vi "OPC.vi"() -> ()   [LabVIEW 2015]
uses:
  <vilib>/Platform/TimedLoop/XDataNode/timing_clust.ctl
  <vilib>/Platform/TimedLoop/XDataNode/nitl_modes.ctl
  <vilib>/Platform/TimedLoop/XDataNode/wakeup.ctl
  Global control/global-opc.vi
  <vilib>/Platform/TimedLoop/XDataNode/XDataNode.xnode
  <vilib>/Platform/TimedLoop/XDataNode/XDNodeRunTimeDep.lvlib
panel:
  out "IP40":T1={"toHMI正常运行"=TRUE, "toHMI设备准备好"=TRUE, "toHMI设备异常"=TRUE, "toHMI刀开关分—状态"=TRUE, "toHMI刀开关合—状态"=TRUE, "toHMI框架电流故障"=TRUE, "toHMI框架电压故障"=TRUE, "toHMII段电压故障"=TRUE, "toHMIII段电压故障"=TRUE, "toHMI装置故障"=TRUE, "toHMIMCB故障"=TRUE, "toHMI刀开关合—完成"=TRUE, "toHMI复位按钮"=TRUE, "toHMI远程"=TRUE, "toHMI本地"=TRUE, "模拟电流框架故障控制"=TRUE, "模拟电压框架故障控制"=TRUE, "模拟I段电压故障控制"=TRUE, "模拟II段电压故障控制"=TRUE, "故障复位控制"=TRUE}
  out "IP30":T2={"toHMI正常运行"=FALSE, "toHMI设备准备好"=FALSE, "toHMI设备异常"=FALSE, "toHMI高断分—状态"=FALSE, "toHMI高断合—状态"=FALSE, "toHMI继保故障信号"=FALSE, "toHMI远方"=FALSE, "toHMI本地"=FALSE, "toHMI旁路合闸—按钮"=FALSE, "toHMI旁路分闸—按钮"=FALSE, "toHMI允许高断合闸—状态"=FALSE, "toHMI旁路合分闸—状态"=FALSE, "1500V电压输出"=0, "高断储能控制"=TRUE, "旁路合闸控制"=TRUE, "旁路分闸控制"=TRUE}
  out "IP20":T3={"toHMI正常运行"=TRUE, "toHMI设备准备好"=TRUE, "toHMI设备异常"=TRUE, "toHMI刀开关合—状态"=TRUE, "toHMI刀开关分—状态"=TRUE, "toHMI刀开关合按钮"=TRUE, "toHMI刀开关分按钮"=TRUE, "toHMI复位按钮"=TRUE, "toHMI远程"=TRUE, "toHMI本地"=TRUE, "toHMI刀闸合—动作"=TRUE, "toHMI刀闸分—动作"=TRUE, "刀开关合闸控制"=TRUE, "刀开关分闸控制"=TRUE, "故障复位控制"=TRUE}
  out "IP10":T4
  out "IP50":T5={"toHMI刀开关合—状态"=TRUE, "toHMI刀开关分—状态"=TRUE, "toHMI刀开关合按钮"=TRUE, "toHMI刀开关分按钮"=TRUE, "toHMI远程"=TRUE, "toHMI本地"=TRUE, "toHMI正常运行"=TRUE, "toHMI设备准备好"=TRUE, "toHMI设备异常"=TRUE, "toHMI刀闸合—动作"=TRUE, "toHMI刀闸分—动作"=TRUE, "toHMI接触轨有压"=TRUE, "刀开关合闸控制"=TRUE, "刀开关分闸控制"=TRUE}
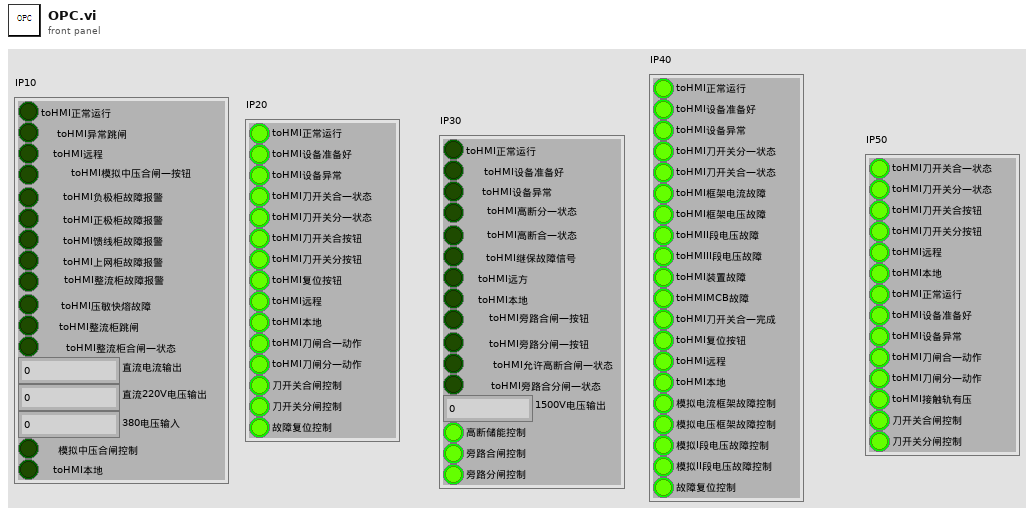
[diagram p1: front panel]
types:
  T1 = cluster{"toHMI正常运行":bool, "toHMI设备准备好":bool, "toHMI设备异常":bool, "toHMI刀开关分—状态":bool, "toHMI刀开关合—状态":bool, "toHMI框架电流故障":bool, "toHMI框架电压故障":bool, "toHMII段电压故障":bool, "toHMIII段电压故障":bool, "toHMI装置故障":bool, "toHMIMCB故障":bool, "toHMI刀开关合—完成":bool, "toHMI复位按钮":bool, "toHMI远程":bool, "toHMI本地":bool, "模拟电流框架故障控制":bool, "模拟电压框架故障控制":bool, "模拟I段电压故障控制":bool, "模拟II段电压故障控制":bool, "故障复位控制":bool}
  T2 = cluster{"toHMI正常运行":bool, "toHMI设备准备好":bool, "toHMI设备异常":bool, "toHMI高断分—状态":bool, "toHMI高断合—状态":bool, "toHMI继保故障信号":bool, "toHMI远方":bool, "toHMI本地":bool, "toHMI旁路合闸—按钮":bool, "toHMI旁路分闸—按钮":bool, "toHMI允许高断合闸—状态":bool, "toHMI旁路合分闸—状态":bool, "1500V电压输出":u32, "高断储能控制":bool, "旁路合闸控制":bool, "旁路分闸控制":bool}
  T3 = cluster{"toHMI正常运行":bool, "toHMI设备准备好":bool, "toHMI设备异常":bool, "toHMI刀开关合—状态":bool, "toHMI刀开关分—状态":bool, "toHMI刀开关合按钮":bool, "toHMI刀开关分按钮":bool, "toHMI复位按钮":bool, "toHMI远程":bool, "toHMI本地":bool, "toHMI刀闸合—动作":bool, "toHMI刀闸分—动作":bool, "刀开关合闸控制":bool, "刀开关分闸控制":bool, "故障复位控制":bool}
  T4 = cluster{"toHMI正常运行":bool, "toHMI异常跳闸":bool, "toHMI远程":bool, "toHMI模拟中压合闸—按钮":bool, "toHMI负极柜故障报警":bool, "toHMI正极柜故障报警":bool, "toHMI馈线柜故障报警":bool, "toHMI上网柜故障报警":bool, "toHMI整流柜故障报警":bool, "toHMI压敏快熔故障":bool, "toHMI整流柜跳闸":bool, "toHMI整流柜合闸—状态":bool, "直流电流输出":u32, "直流220V电压输出":u32, "380电压输入":u32, "模拟中压合闸控制":bool, "toHMI本地":bool}
  T5 = cluster{"toHMI刀开关合—状态":bool, "toHMI刀开关分—状态":bool, "toHMI刀开关合按钮":bool, "toHMI刀开关分按钮":bool, "toHMI远程":bool, "toHMI本地":bool, "toHMI正常运行":bool, "toHMI设备准备好":bool, "toHMI设备异常":bool, "toHMI刀闸合—动作":bool, "toHMI刀闸分—动作":bool, "toHMI接触轨有压":bool, "刀开关合闸控制":bool, "刀开关分闸控制":bool}
  T6 = typedef "XDNodeRunTimeDep.lvlib/timing_clust.ctl" = cluster{"Expected End [f-1]":u64, "Actual End [f-1]":u64, "Finished Late? [f-1]":bool, "Expected End [i-1]":u64, "Actual End [i-1]":u64, "Finished Late? [i-1]":bool, "Expected Start [i]":u64, "Actual Start [i]":u64, "Expected Start [f]":u64, "Actual Start [f]":u64, "Source Name":string, "Structure Name":string, "Period":i64, "Deadline":i64, "Offset":i64, "Start":i64, "Priority":i32, "Timeout":i32, "Mode":T7, "Wakeup Reason":T8, "Error":errorcluster, "Source Type":string, "Secondary Source Type":string, "Global End Time":u64, "Global Start Time":u64, "Frame Duration":u64, "Iteration Duration":u64, "Assigned CPU":i32, "I/O Scan Engine Mode":u32}
  T7 = typedef "XDNodeRunTimeDep.lvlib/nitl_modes.ctl" = enum32{"No Change", "Process missed periods, maintain original phase", "Discard missed periods, maintain original phase", "Process missed periods, ignore original phase", "Discard missed periods, ignore original phase"}
  T8 = typedef "XDNodeRunTimeDep.lvlib/wakeup.ctl" = enum32{"Normal", "Aborted", "Asynchronous wakeup", "Timing source error", "Timed loop error", "Timeout"}
  T9 = cluster{bool, bool, bool, bool, bool, bool, bool, bool, bool, bool, bool, bool, bool, bool, bool}
  T10 = cluster{bool, bool, bool, bool, bool, bool, bool, bool, bool, bool, bool, bool, u32, bool, bool, bool}
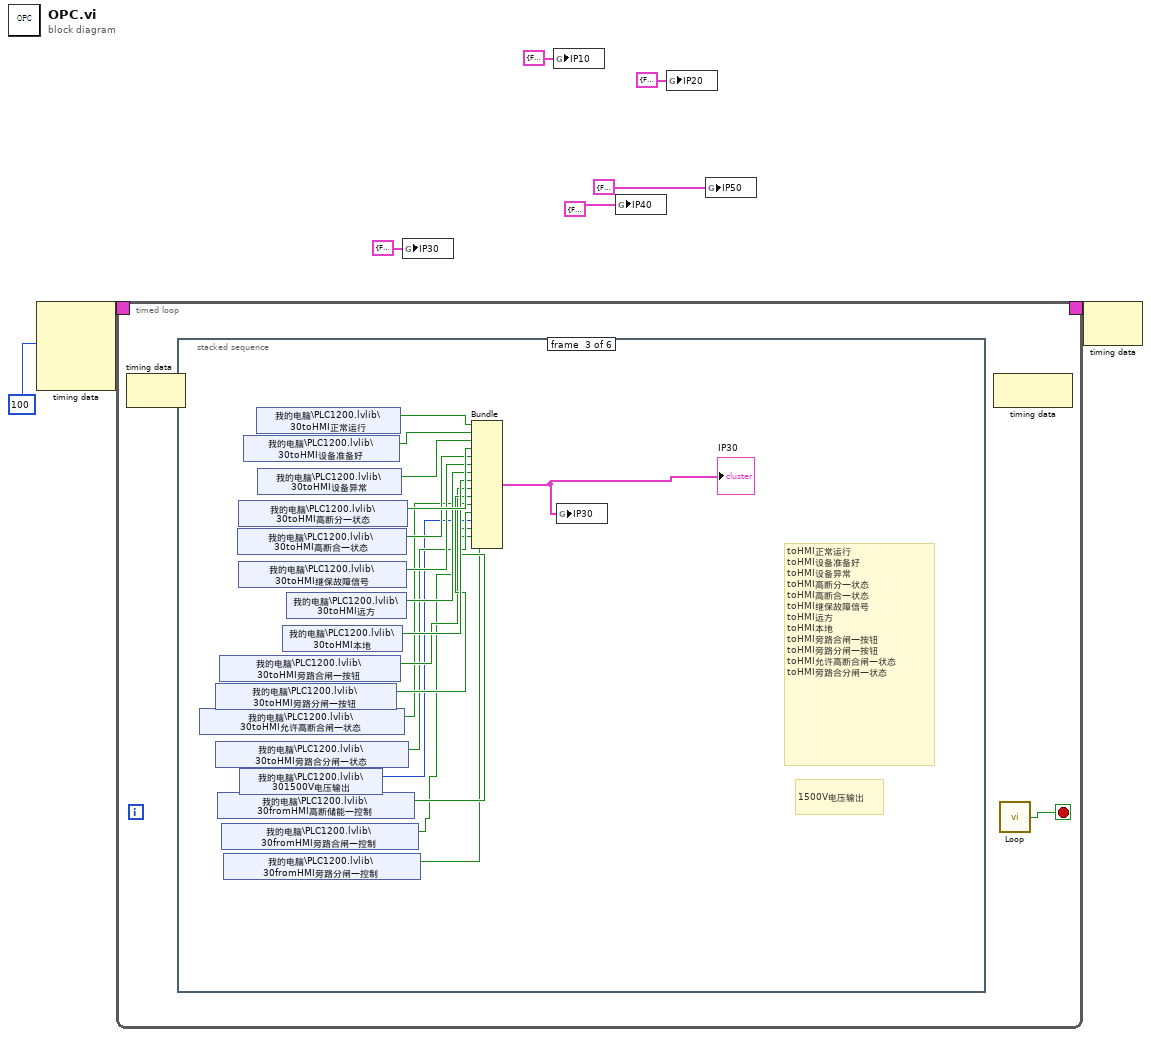
[diagram p0: block diagram]
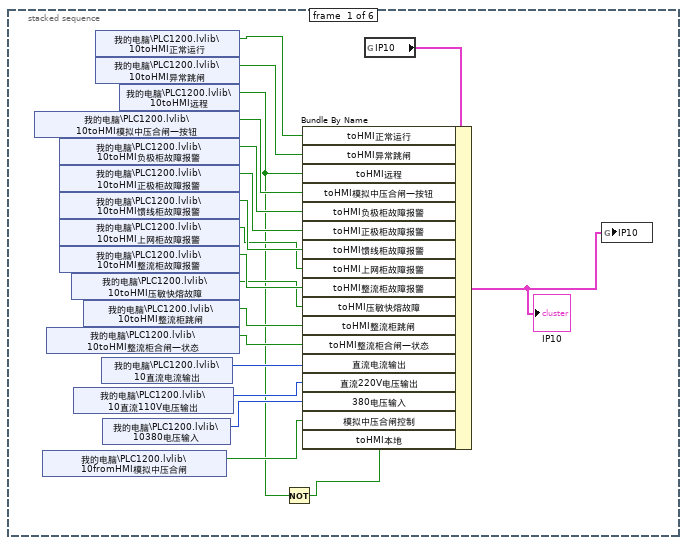
[diagram p2: hidden frame]
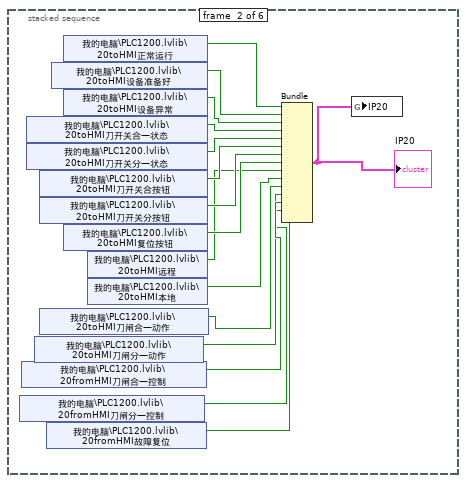
[diagram p3: hidden frame]
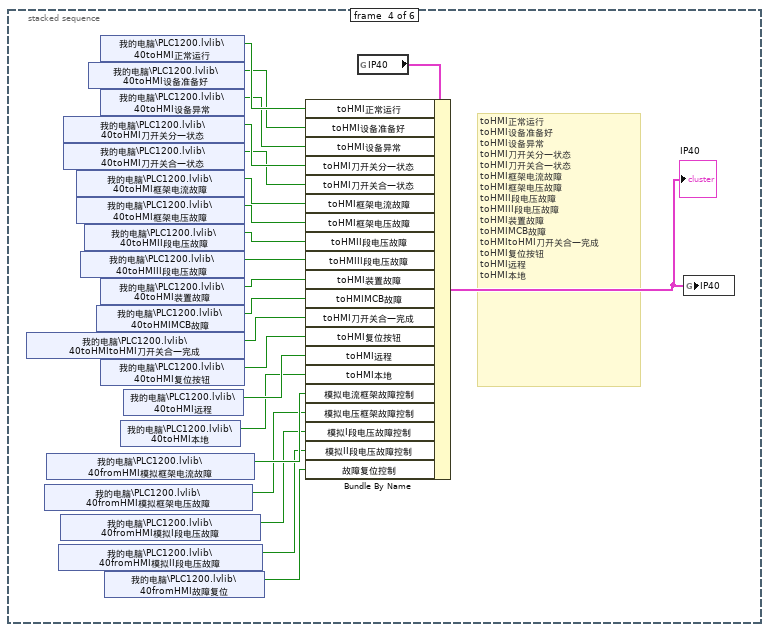
[diagram p4: hidden frame]
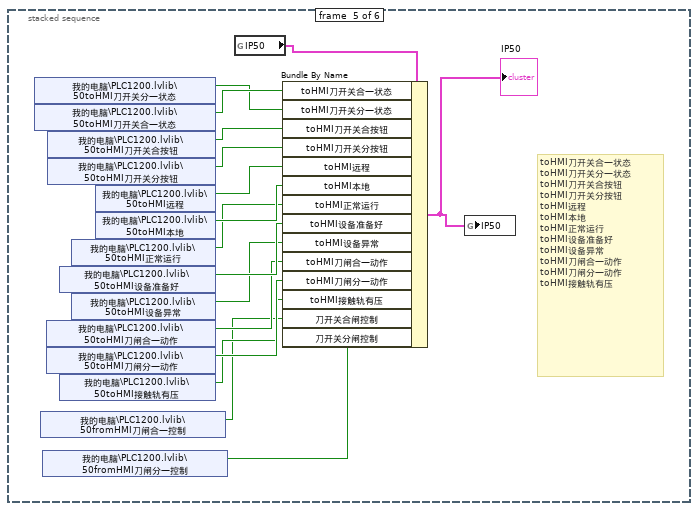
[diagram p5: hidden frame]
diagram:
  n1 = node-c288(i64 100 ("周期")) -> (w8:T6)  [unwired: 3 in]
  n2 = timed-loop {
    timing: w8 -> [_]
    timing-out: [_] -> w7
    stop <- w9 stop-if-true
    # "IP192.168.0.10"
    n3 = node-c288() -> ()  [unwired: 1 in, 1 out]
    n4 = stacked-sequence {
      frame #0 {
        n5 = shared-variable "我的电脑\\PLC1200.lvlib\\10toHMI模拟中压合闸—按钮"() -> (w25:bool)  [unwired: 1 in, 1 out]
        n6 = shared-variable "我的电脑\\PLC1200.lvlib\\10fromHMI模拟中压合闸"() -> (w13:bool)  [unwired: 1 in, 1 out]
        n7 = shared-variable "我的电脑\\PLC1200.lvlib\\10toHMI整流柜合闸—状态"() -> (w17:bool)  [unwired: 1 in, 1 out]
        n8 = shared-variable "我的电脑\\PLC1200.lvlib\\10toHMI负极柜故障报警"() -> (w24:bool)  [unwired: 1 in, 1 out]
        n9 = shared-variable "我的电脑\\PLC1200.lvlib\\10toHMI正极柜故障报警"() -> (w23:bool)  [unwired: 1 in, 1 out]
        n10 = shared-variable "我的电脑\\PLC1200.lvlib\\10toHMI馈线柜故障报警"() -> (w22:bool)  [unwired: 1 in, 1 out]
        n11 = shared-variable "我的电脑\\PLC1200.lvlib\\10toHMI上网柜故障报警"() -> (w21:bool)  [unwired: 1 in, 1 out]
        n12 = shared-variable "我的电脑\\PLC1200.lvlib\\10toHMI整流柜故障报警"() -> (w20:bool)  [unwired: 1 in, 1 out]
        n13 = shared-variable "我的电脑\\PLC1200.lvlib\\10toHMI压敏快熔故障"() -> (w19:bool)  [unwired: 1 in, 1 out]
        n14 = shared-variable "我的电脑\\PLC1200.lvlib\\10直流110V电压输出"() -> (w15:u32)  [unwired: 1 in, 1 out]
        n15 = shared-variable "我的电脑\\PLC1200.lvlib\\10toHMI整流柜跳闸"() -> (w18:bool)  [unwired: 1 in, 1 out]
        n16 = shared-variable "我的电脑\\PLC1200.lvlib\\10toHMI正常运行"() -> (w27:bool)  [unwired: 1 in, 1 out]
        n17 = shared-variable "我的电脑\\PLC1200.lvlib\\10toHMI异常跳闸"() -> (w26:bool)  [unwired: 1 in, 1 out]
        n18 = shared-variable "我的电脑\\PLC1200.lvlib\\10直流电流输出"() -> (w16:u32)  [unwired: 1 in, 1 out]
        n19 = shared-variable "我的电脑\\PLC1200.lvlib\\10380电压输入"() -> (w14:u32)  [unwired: 1 in, 1 out]
        n20 = shared-variable "我的电脑\\PLC1200.lvlib\\10toHMI远程"() -> (w11:bool)  [unwired: 1 in, 1 out]
        n21 = Not(x=w11) -> (.not. x?=w10:bool)
        n22 = global read "global-opc.vi" "IP10"() -> (w28:T4)
        n23 = Bundle By Name(cluster=w28, "toHMI正常运行"=w27, "toHMI异常跳闸"=w26, "toHMI远程"=w11, "toHMI模拟中压合闸—按钮"=w25, "toHMI负极柜故障报警"=w24, "toHMI正极柜故障报警"=w23, "toHMI馈线柜故障报警"=w22, "toHMI上网柜故障报警"=w21, "toHMI整流柜故障报警"=w20, "toHMI压敏快熔故障"=w19, "toHMI整流柜跳闸"=w18, "toHMI整流柜合闸—状态"=w17, "直流电流输出"=w16, "直流220V电压输出"=w15, "380电压输入"=w14, "模拟中压合闸控制"=w13, "toHMI本地"=w10) -> (w12:T4)
        "IP10" <- w12
        n24 = global write "global-opc.vi" "IP10"(w12) -> ()
      }
      frame #1 {
        n25 = shared-variable "我的电脑\\PLC1200.lvlib\\20fromHMI刀闸分—控制"() -> (w32:bool)  [unwired: 1 in, 1 out]
        n26 = shared-variable "我的电脑\\PLC1200.lvlib\\20fromHMI刀闸合—控制"() -> (w33:bool)  [unwired: 1 in, 1 out]
        n27 = shared-variable "我的电脑\\PLC1200.lvlib\\20toHMI刀开关合—状态"() -> (w44:bool)  [unwired: 1 in, 1 out]
        n28 = shared-variable "我的电脑\\PLC1200.lvlib\\20toHMI刀开关分—状态"() -> (w43:bool)  [unwired: 1 in, 1 out]
        n29 = shared-variable "我的电脑\\PLC1200.lvlib\\20toHMI刀闸分—动作"() -> (w30:bool)  [unwired: 1 in, 1 out]
        n30 = shared-variable "我的电脑\\PLC1200.lvlib\\20toHMI刀开关合按钮"() -> (w42:bool)  [unwired: 1 in, 1 out]
        n31 = shared-variable "我的电脑\\PLC1200.lvlib\\20toHMI刀开关分按钮"() -> (w41:bool)  [unwired: 1 in, 1 out]
        n32 = shared-variable "我的电脑\\PLC1200.lvlib\\20toHMI刀闸合—动作"() -> (w29:bool)  [unwired: 1 in, 1 out]
        n33 = shared-variable "我的电脑\\PLC1200.lvlib\\20fromHMI故障复位"() -> (w31:bool)  [unwired: 1 in, 1 out]
        n34 = shared-variable "我的电脑\\PLC1200.lvlib\\20toHMI设备准备好"() -> (w36:bool)  [unwired: 1 in, 1 out]
        n35 = shared-variable "我的电脑\\PLC1200.lvlib\\20toHMI正常运行"() -> (w37:bool)  [unwired: 1 in, 1 out]
        n36 = shared-variable "我的电脑\\PLC1200.lvlib\\20toHMI设备异常"() -> (w35:bool)  [unwired: 1 in, 1 out]
        n37 = shared-variable "我的电脑\\PLC1200.lvlib\\20toHMI复位按钮"() -> (w40:bool)  [unwired: 1 in, 1 out]
        n38 = shared-variable "我的电脑\\PLC1200.lvlib\\20toHMI远程"() -> (w39:bool)  [unwired: 1 in, 1 out]
        n39 = shared-variable "我的电脑\\PLC1200.lvlib\\20toHMI本地"() -> (w38:bool)  [unwired: 1 in, 1 out]
        n40 = Bundle(w37, w36, w35, w44, w43, w42, w41, w40, w39, w38, w29, w30, w33, w32, w31) -> (w34:T9)  [unwired: 1 in]
        "IP20" <- w34
        n41 = global write "global-opc.vi" "IP20"(w34) -> ()
      }
      frame #2 {
        # "1500V电压输出"
        # "toHMI正常运行\ntoHMI设备准备好\ntoHMI设备异常\ntoHMI高断分—状态\ntoHMI高断合—状态\ntoHMI继保故障信号\ntoHMI远方\ntoHMI本地\ntoHMI旁路合闸—按钮\ntoHMI旁路分闸—按钮\ntoHMI允许高断合闸—状态\ntoHMI旁路合分闸—状态"
        n42 = shared-variable "我的电脑\\PLC1200.lvlib\\30toHMI允许高断合闸—状态"() -> (w51:bool)  [unwired: 1 in, 1 out]
        n43 = shared-variable "我的电脑\\PLC1200.lvlib\\30toHMI旁路分闸—按钮"() -> (w53:bool)  [unwired: 1 in, 1 out]
        n44 = shared-variable "我的电脑\\PLC1200.lvlib\\30toHMI旁路合分闸—状态"() -> (w50:bool)  [unwired: 1 in, 1 out]
        n45 = shared-variable "我的电脑\\PLC1200.lvlib\\30fromHMI高断储能—控制"() -> (w47:bool)  [unwired: 1 in, 1 out]
        n46 = shared-variable "我的电脑\\PLC1200.lvlib\\30toHMI旁路合闸—按钮"() -> (w52:bool)  [unwired: 1 in, 1 out]
        n47 = shared-variable "我的电脑\\PLC1200.lvlib\\30fromHMI旁路合闸—控制"() -> (w46:bool)  [unwired: 1 in, 1 out]
        n48 = shared-variable "我的电脑\\PLC1200.lvlib\\30fromHMI旁路分闸—控制"() -> (w45:bool)  [unwired: 1 in, 1 out]
        n49 = shared-variable "我的电脑\\PLC1200.lvlib\\30toHMI高断合—状态"() -> (w57:bool)  [unwired: 1 in, 1 out]
        n50 = shared-variable "我的电脑\\PLC1200.lvlib\\30toHMI高断分—状态"() -> (w58:bool)  [unwired: 1 in, 1 out]
        n51 = shared-variable "我的电脑\\PLC1200.lvlib\\30toHMI继保故障信号"() -> (w56:bool)  [unwired: 1 in, 1 out]
        n52 = shared-variable "我的电脑\\PLC1200.lvlib\\301500V电压输出"() -> (w49:u32)  [unwired: 1 in, 1 out]
        n53 = shared-variable "我的电脑\\PLC1200.lvlib\\30toHMI设备准备好"() -> (w60:bool)  [unwired: 1 in, 1 out]
        n54 = shared-variable "我的电脑\\PLC1200.lvlib\\30toHMI正常运行"() -> (w61:bool)  [unwired: 1 in, 1 out]
        n55 = shared-variable "我的电脑\\PLC1200.lvlib\\30toHMI设备异常"() -> (w59:bool)  [unwired: 1 in, 1 out]
        n56 = shared-variable "我的电脑\\PLC1200.lvlib\\30toHMI本地"() -> (w54:bool)  [unwired: 1 in, 1 out]
        n57 = shared-variable "我的电脑\\PLC1200.lvlib\\30toHMI远方"() -> (w55:bool)  [unwired: 1 in, 1 out]
        n58 = Bundle(w61, w60, w59, w58, w57, w56, w55, w54, w52, w53, w51, w50, w49, w47, w46, w45) -> (w48:T10)  [unwired: 1 in]
        "IP30" <- w48
        n59 = global write "global-opc.vi" "IP30"(w48) -> ()
      }
      frame #3 {
        # "toHMI正常运行\ntoHMI设备准备好\ntoHMI设备异常\ntoHMI刀开关分—状态\ntoHMI刀开关合—状态\ntoHMI框架电流故障\ntoHMI框架电压故障\ntoHMII段电压故障\ntoHMIII段电压故障\ntoHMI装置故障\ntoHMIMCB故障\ntoHMItoHMI刀开关合—完成\ntoHMI复位按钮\ntoHMI远程\ntoHMI本地"
        n60 = shared-variable "我的电脑\\PLC1200.lvlib\\40toHMItoHMI刀开关合—完成"() -> (w72:bool)  [unwired: 1 in, 1 out]
        n61 = shared-variable "我的电脑\\PLC1200.lvlib\\40fromHMI模拟框架电压故障"() -> (w65:bool)  [unwired: 1 in, 1 out]
        n62 = shared-variable "我的电脑\\PLC1200.lvlib\\40fromHMI模拟框架电流故障"() -> (w66:bool)  [unwired: 1 in, 1 out]
        n63 = shared-variable "我的电脑\\PLC1200.lvlib\\40fromHMI模拟II段电压故障"() -> (w63:bool)  [unwired: 1 in, 1 out]
        n64 = shared-variable "我的电脑\\PLC1200.lvlib\\40fromHMI模拟I段电压故障"() -> (w64:bool)  [unwired: 1 in, 1 out]
        n65 = shared-variable "我的电脑\\PLC1200.lvlib\\40toHMI刀开关分—状态"() -> (w80:bool)  [unwired: 1 in, 1 out]
        n66 = shared-variable "我的电脑\\PLC1200.lvlib\\40toHMI刀开关合—状态"() -> (w79:bool)  [unwired: 1 in, 1 out]
        n67 = shared-variable "我的电脑\\PLC1200.lvlib\\40toHMI框架电流故障"() -> (w78:bool)  [unwired: 1 in, 1 out]
        n68 = shared-variable "我的电脑\\PLC1200.lvlib\\40toHMI框架电压故障"() -> (w77:bool)  [unwired: 1 in, 1 out]
        n69 = shared-variable "我的电脑\\PLC1200.lvlib\\40toHMIII段电压故障"() -> (w75:bool)  [unwired: 1 in, 1 out]
        n70 = shared-variable "我的电脑\\PLC1200.lvlib\\40toHMII段电压故障"() -> (w76:bool)  [unwired: 1 in, 1 out]
        n71 = shared-variable "我的电脑\\PLC1200.lvlib\\40toHMI设备准备好"() -> (w82:bool)  [unwired: 1 in, 1 out]
        n72 = shared-variable "我的电脑\\PLC1200.lvlib\\40toHMIMCB故障"() -> (w73:bool)  [unwired: 1 in, 1 out]
        n73 = shared-variable "我的电脑\\PLC1200.lvlib\\40toHMI正常运行"() -> (w83:bool)  [unwired: 1 in, 1 out]
        n74 = shared-variable "我的电脑\\PLC1200.lvlib\\40toHMI设备异常"() -> (w81:bool)  [unwired: 1 in, 1 out]
        n75 = shared-variable "我的电脑\\PLC1200.lvlib\\40toHMI装置故障"() -> (w74:bool)  [unwired: 1 in, 1 out]
        n76 = shared-variable "我的电脑\\PLC1200.lvlib\\40toHMI复位按钮"() -> (w71:bool)  [unwired: 1 in, 1 out]
        n77 = shared-variable "我的电脑\\PLC1200.lvlib\\40fromHMI故障复位"() -> (w62:bool)  [unwired: 1 in, 1 out]
        n78 = shared-variable "我的电脑\\PLC1200.lvlib\\40toHMI本地"() -> (w69:bool)  [unwired: 1 in, 1 out]
        n79 = shared-variable "我的电脑\\PLC1200.lvlib\\40toHMI远程"() -> (w70:bool)  [unwired: 1 in, 1 out]
        n80 = global read "global-opc.vi" "IP40"() -> (w68:T1)
        n81 = Bundle By Name(cluster=w68, "toHMI正常运行"=w83, "toHMI设备准备好"=w82, "toHMI设备异常"=w81, "toHMI刀开关分—状态"=w80, "toHMI刀开关合—状态"=w79, "toHMI框架电流故障"=w78, "toHMI框架电压故障"=w77, "toHMII段电压故障"=w76, "toHMIII段电压故障"=w75, "toHMI装置故障"=w74, "toHMIMCB故障"=w73, "toHMI刀开关合—完成"=w72, "toHMI复位按钮"=w71, "toHMI远程"=w70, "toHMI本地"=w69, "模拟电流框架故障控制"=w66, "模拟电压框架故障控制"=w65, "模拟I段电压故障控制"=w64, "模拟II段电压故障控制"=w63, "故障复位控制"=w62) -> (w67:T1)
        "IP40" <- w67
        n82 = global write "global-opc.vi" "IP40"(w67) -> ()
      }
      frame #4 {
        # "toHMI刀开关合—状态\ntoHMI刀开关分—状态\ntoHMI刀开关合按钮\ntoHMI刀开关分按钮\ntoHMI远程\ntoHMI本地\ntoHMI正常运行\ntoHMI设备准备好\ntoHMI设备异常\ntoHMI刀闸合—动作\ntoHMI刀闸分—动作\ntoHMI接触轨有压"
        n83 = shared-variable "我的电脑\\PLC1200.lvlib\\50toHMI刀开关分—状态"() -> (w84:bool)  [unwired: 1 in, 1 out]
        n84 = shared-variable "我的电脑\\PLC1200.lvlib\\50toHMI刀开关合—状态"() -> (w85:bool)  [unwired: 1 in, 1 out]
        n85 = shared-variable "我的电脑\\PLC1200.lvlib\\50fromHMI刀闸合—控制"() -> (w87:bool)  [unwired: 1 in, 1 out]
        n86 = shared-variable "我的电脑\\PLC1200.lvlib\\50fromHMI刀闸分—控制"() -> (w86:bool)  [unwired: 1 in, 1 out]
        n87 = shared-variable "我的电脑\\PLC1200.lvlib\\50toHMI刀闸合—动作"() -> (w92:bool)  [unwired: 1 in, 1 out]
        n88 = shared-variable "我的电脑\\PLC1200.lvlib\\50toHMI刀闸分—动作"() -> (w91:bool)  [unwired: 1 in, 1 out]
        n89 = shared-variable "我的电脑\\PLC1200.lvlib\\50toHMI刀开关合按钮"() -> (w99:bool)  [unwired: 1 in, 1 out]
        n90 = shared-variable "我的电脑\\PLC1200.lvlib\\50toHMI刀开关分按钮"() -> (w98:bool)  [unwired: 1 in, 1 out]
        n91 = shared-variable "我的电脑\\PLC1200.lvlib\\50toHMI设备准备好"() -> (w94:bool)  [unwired: 1 in, 1 out]
        n92 = shared-variable "我的电脑\\PLC1200.lvlib\\50toHMI接触轨有压"() -> (w90:bool)  [unwired: 1 in, 1 out]
        n93 = shared-variable "我的电脑\\PLC1200.lvlib\\50toHMI正常运行"() -> (w95:bool)  [unwired: 1 in, 1 out]
        n94 = shared-variable "我的电脑\\PLC1200.lvlib\\50toHMI设备异常"() -> (w93:bool)  [unwired: 1 in, 1 out]
        n95 = shared-variable "我的电脑\\PLC1200.lvlib\\50toHMI远程"() -> (w97:bool)  [unwired: 1 in, 1 out]
        n96 = shared-variable "我的电脑\\PLC1200.lvlib\\50toHMI本地"() -> (w96:bool)  [unwired: 1 in, 1 out]
        n97 = global read "global-opc.vi" "IP50"() -> (w89:T5)
        n98 = Bundle By Name(cluster=w89, "toHMI刀开关合—状态"=w85, "toHMI刀开关分—状态"=w84, "toHMI刀开关合按钮"=w99, "toHMI刀开关分按钮"=w98, "toHMI远程"=w97, "toHMI本地"=w96, "toHMI正常运行"=w95, "toHMI设备准备好"=w94, "toHMI设备异常"=w93, "toHMI刀闸合—动作"=w92, "toHMI刀闸分—动作"=w91, "toHMI接触轨有压"=w90, "刀开关合闸控制"=w87, "刀开关分闸控制"=w86) -> (w88:T5)
        "IP50" <- w88
        n99 = global write "global-opc.vi" "IP50"(w88) -> ()
      }
      frame #5 {
      }
    }
    n100 = node-c288() -> ()  [unwired: 1 in, 1 out]
    n101 = call "Loop.vi"() -> ("Loop Out"=w9:bool)  [unwired: 5 in]
  }
  n102 = global write "global-opc.vi" "IP30"(T2 {"toHMI正常运行"=FALSE, "toHMI设备准备好"=FALSE, "toHMI设备异常"=FALSE, "toHMI高断分—状态"=FALSE, "toHMI高断合—状态"=FALSE, "toHMI继保故障信号"=FALSE, "toHMI远方"=FALSE, "toHMI本地"=FALSE, "toHMI旁路合闸—按钮"=FALSE, "toHMI旁路分闸—按钮"=FALSE, "toHMI允许高断合闸—状态"=FALSE, "toHMI旁路合分闸—状态"=FALSE, "1500V电压输出"=0, "高断储能控制"=FALSE, "旁路合闸控制"=FALSE, "旁路分闸控制"=FALSE} ("IP30")) -> ()
  n103 = global write "global-opc.vi" "IP10"(T4 {"toHMI正常运行"=FALSE, "toHMI异常跳闸"=FALSE, "toHMI远程"=FALSE, "toHMI模拟中压合闸—按钮"=FALSE, "toHMI负极柜故障报警"=FALSE, "toHMI正极柜故障报警"=FALSE, "toHMI馈线柜故障报警"=FALSE, "toHMI上网柜故障报警"=FALSE, "toHMI整流柜故障报警"=FALSE, "toHMI压敏快熔故障"=FALSE, "toHMI整流柜跳闸"=FALSE, "toHMI整流柜合闸—状态"=FALSE, "直流电流输出"=0, "直流220V电压输出"=0, "380电压输入"=0, "模拟中压合闸控制"=FALSE, "toHMI本地"=FALSE} ("IP10")) -> ()
  n104 = global write "global-opc.vi" "IP40"(T1 {"toHMI正常运行"=FALSE, "toHMI设备准备好"=FALSE, "toHMI设备异常"=FALSE, "toHMI刀开关分—状态"=FALSE, "toHMI刀开关合—状态"=FALSE, "toHMI框架电流故障"=FALSE, "toHMI框架电压故障"=FALSE, "toHMII段电压故障"=FALSE, "toHMIII段电压故障"=FALSE, "toHMI装置故障"=FALSE, "toHMIMCB故障"=FALSE, "toHMI刀开关合—完成"=FALSE, "toHMI复位按钮"=FALSE, "toHMI远程"=FALSE, "toHMI本地"=FALSE, "模拟电流框架故障控制"=FALSE, "模拟电压框架故障控制"=FALSE, "模拟I段电压故障控制"=FALSE, "模拟II段电压故障控制"=FALSE, "故障复位控制"=FALSE} ("IP40")) -> ()
  n105 = global write "global-opc.vi" "IP20"(T3 {"toHMI正常运行"=FALSE, "toHMI设备准备好"=FALSE, "toHMI设备异常"=FALSE, "toHMI刀开关合—状态"=FALSE, "toHMI刀开关分—状态"=FALSE, "toHMI刀开关合按钮"=FALSE, "toHMI刀开关分按钮"=FALSE, "toHMI复位按钮"=FALSE, "toHMI远程"=FALSE, "toHMI本地"=FALSE, "toHMI刀闸合—动作"=FALSE, "toHMI刀闸分—动作"=FALSE, "刀开关合闸控制"=FALSE, "刀开关分闸控制"=FALSE, "故障复位控制"=FALSE} ("IP20")) -> ()
  n106 = global write "global-opc.vi" "IP50"(T5 {"toHMI刀开关合—状态"=FALSE, "toHMI刀开关分—状态"=FALSE, "toHMI刀开关合按钮"=FALSE, "toHMI刀开关分按钮"=FALSE, "toHMI远程"=FALSE, "toHMI本地"=FALSE, "toHMI正常运行"=FALSE, "toHMI设备准备好"=FALSE, "toHMI设备异常"=FALSE, "toHMI刀闸合—动作"=FALSE, "toHMI刀闸分—动作"=FALSE, "toHMI接触轨有压"=FALSE, "刀开关合闸控制"=FALSE, "刀开关分闸控制"=FALSE} ("IP50")) -> ()
  n107 = node-c288(w7) -> ()  [unwired: 1 out]
